vi "MGI Path To Symbolic.vi"(10 "Path":path) -> (1 "Symbolic Folder":T1, 2 "Symbolic?":bool, 3 "Symbolic Path":path)   [LabVIEW 2020]
doc: "Build an symbolic path from the specified Path. A Symbolic path contains an initial fake directory such as \"<Desktop>\". If the specified path doesn't map to any symbolic paths, then output the specified path as the symbolic path.\n\nAuthored by Shawn Walpole\nsupport@mooregoodideas.com\nwww.mooregoodideas.com\n\nCopyright (c) 2013, Moore Good Ideas, Inc.\n\nAll rights reserved.\n\nRedistribution and use in source and binary forms, with or without modification, are permitted provided that the following conditions are met:\n\n * Redistributions of source code must retain the above copyright notice, this list of conditions and the following disclaimer.\n * Redistributions in binary form must reproduce the above copyright notice, this list of conditions and the following disclaimer in the documentation and/or other materials provided with the distribution.\n * Neither the name of Moore Good Ideas, Inc. nor the names of its contributors may be used to endorse or promote products derived from this software without specific prior written permission.\n\nTHIS SOFTWARE IS PROVIDED BY THE COPYRIGHT HOLDERS AND CONTRIBUTORS \"AS IS\" AND ANY EXPRESS OR IMPLIED WARRANTIES, INCLUDING, BUT NOT LIMITED TO, THE IMPLIED WARRANTIES OF MERCHANTABILITY AND FITNESS FOR A PARTICULAR PURPOSE ARE DISCLAIMED. IN NO EVENT SHALL THE COPYRIGHT OWNER OR CONTRIBUTORS BE LIABLE FOR ANY DIRECT, INDIRECT, INCIDENTAL, SPECIAL, EXEMPLARY, OR CONSEQUENTIAL DAMAGES (INCLUDING, BUT NOT LIMITED TO, PROCUREMENT OF SUBSTITUTE GOODS OR SERVICES; LOSS OF USE, DATA, OR PROFITS; OR BUSINESS INTERRUPTION) HOWEVER CAUSED AND ON ANY THEORY OF LIABILITY, WHETHER IN CONTRACT, STRICT LIABILITY, OR TORT (INCLUDING NEGLIGENCE OR OTHERWISE) ARISING IN ANY WAY OUT OF THE USE OF THIS SOFTWARE, EVEN IF ADVISED OF THE POSSIBILITY OF SUCH DAMAGE."
uses:
  <userlib>/_MGI/File/MGI Windows Folder Enum.ctl
  <vilib>/Utility/VariantDataType/VariantType.lvlib
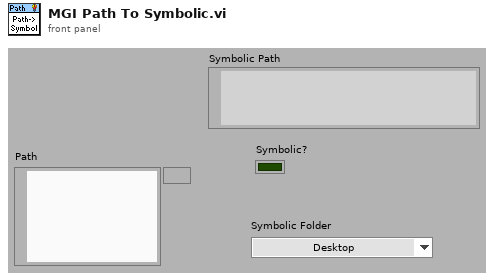
[diagram p1: front panel]
types:
  T1 = typedef "MGI Windows Folder Enum.ctl" = enum32{"Desktop", "Err<Internet>", "Programs", "Err<Controls>", "Err<Printers>", "Personal (MyDocuments)", "Favorites", "Startup", "Recent", "SendTo", "Err<RecycleBin>", "StartMenu", "Err<MyDocuments>", "MyMusic", "MyVideo", "Err<0x000F>", "DesktopDirectory", "Err<Drives>", "Err<Network>", "NetHood", "Fonts", "Templates", "CommonStartMenu", "CommonPrograms", "CommonStartup", "CommonDesktopDirectory", "AppData", "PrintHood", "LocalAppData", "Err<AltStartup>", "Err<CommonAltStartup>", "CommonFavorites", "InternetCache", "Cookies", "History", "CommonAppData", "Windows", "System", "ProgramFiles", "MyPictures", "Profile", "System32", "Err<0x002A>", "ProgramFilesCommon", "Err<0x002C>", "CommonTemplates", "CommonDocuments", "CommonAdminTools", "AdminTools"}
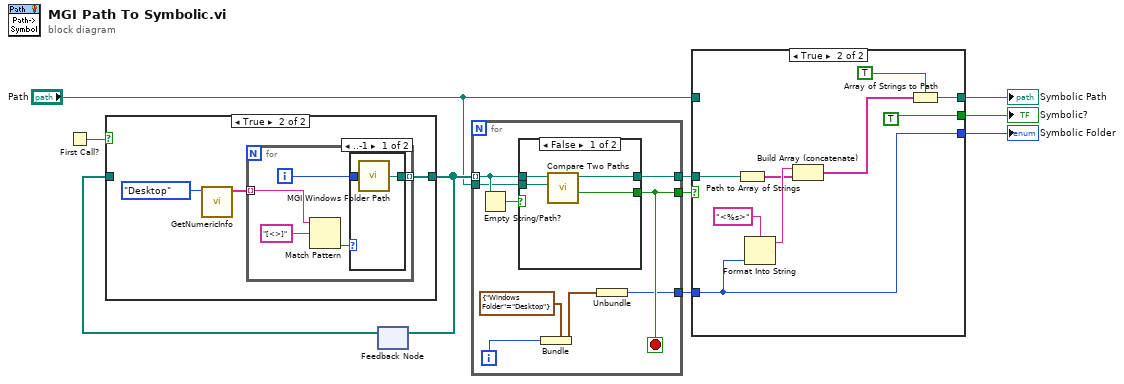
[diagram p0: block diagram]
diagram:
  n1 = First Call?() -> (First Call?: T/F=w10:bool)
  n2 = feedback #1() -> (w9:path[])  [unwired: 1 in]
  n3 = case shown="True" w10 {
    tunnel: [w11 w13] -> w8
    tunnel: w9 -> [w11 _]
    frame False {
    }
    frame True {
      n4 = call <vilib>:"GetNumericInfo.vi"("Variant"=MGI_Windows_Folder_Enum."Desktop" ("Windows Folder")) -> ("EnumNames"=w14:string[])  [unwired: 7 in, 3 out]
      n5 = for {
        tunnel: w14 -> [w19] mode=indexing
        tunnel: [w15] -> w13 mode=indexing
        i -> [w17]
        n6 = Match Pattern(string=w19, regular expression="[<>]") -> (offset past match=w16:i32)  [unwired: 1 in, 3 out]
        n7 = case shown="..-1" w16 {
          tunnel: w17 -> [w21 _]
          tunnel: [w20 _] -> w15
          frame ..-1 {
            n8 = call <userlib>:"MGI Windows Folder Path.vi"("Windows Folder"=w21) -> ("Path"=w20:path)
          }
          frame 0.. {
          }
        }
      }
    }
  }
  n9 = feedback-in #1(w8) -> ()
  n10 = for {
    tunnel: w8 -> [w30] mode=indexing
    tunnel: "Path" -> [w29]
    tunnel: [w27] -> w6
    tunnel: [w26] -> w7
    tunnel: [w22] -> w3
    i -> [w24]
    stop <- w26 stop-if-true
    n11 = Empty String/Path?(string/path=w30) -> (empty?=w28:bool)
    n12 = case shown="False" w28 {
      tunnel: w30 -> [w34 _]
      tunnel: w29 -> [w33 _]
      tunnel: [w32 _] -> w26
      tunnel: [w31 _] -> w27
      frame False {
        n13 = call <vilib>:"Compare Two Paths.vi"("Path 2"=w33, "Path 1"=w34) -> ("Path 2 Relative to Path 1?"=w32:bool, "Relative Path from 1 to 2"=w31:path)  [unwired: 6 in, 2 out]
      }
      frame True {
      }
    }
    n14 = Bundle(cluster=cluster{"Windows Folder":T1} {"Windows Folder"=enum."Desktop"}, "Windows Folder"=w24) -> (w23:cluster{"Windows Folder":T1})
    n15 = Unbundle(w23) -> ("Windows Folder"=w22:T1)
  }
  n16 = case shown="True" w7 {
    tunnel: w6 -> [_ w41]
    tunnel: "Path" -> [w35 _]
    tunnel: [w35 w43] -> w4
    tunnel: w3 -> [_ w37]
    tunnel: [_ w37] -> w2
    tunnel: [_ TRUE ("relative")] -> w1
    frame False {
    }
    frame True {
      n17 = Path to Array of Strings(0:w41) -> (2:w39:string[])  [unwired: 1 out]
      n18 = Format Into String(format string="<%s>", w37) -> (resulting string=w40:string)  [unwired: 2 in, 1 out]
      n19 = Build Array (concatenate)(w40, w39) -> (w38:string[])
      n20 = Array of Strings to Path(0:w38, 1:TRUE ("relative")) -> (2:w43:path)
    }
  }
  "Symbolic Path" <- w4
  "Symbolic?" <- w1
  "Symbolic Folder" <- w2
